vi "Send Count To Caller.vi"(8 "error in (no error)":errorcluster, 10 "Counter":u8, 11 "Counter in":refnum<class "Counter.lvclass">) -> (0 "error out":errorcluster, 3 "Counter out":refnum<class "Counter.lvclass">)   [LabVIEW 2020, in "Counter.lvlib" / "Counter.lvclass"]
uses:
  Counter.lvclass
  C:/Program Files (x86)/National Instruments/LabVIEW 2020/vi.lib/ActorFramework/Actor/Actor.lvclass
  <vilib>/ActorFramework/Actor/Actor.lvclass/Actor.ctl
  Digital Acquisition Messages/Update Data Msg/Update Data Msg.lvclass/Update Data Msg.ctl
  <vilib>/ActorFramework/Message Enqueuer/Message Enqueuer.lvclass/Message Enqueuer.ctl
  <vilib>/ActorFramework/Message Enqueuer/Enqueue.vi
  Digital Acquisition Messages/Update Data Msg/Update Data Msg.lvclass
  C:/Program Files (x86)/National Instruments/LabVIEW 2020/vi.lib/ActorFramework/Message/Message.lvclass
  <vilib>/ActorFramework/Message Priority Queue/Priority Enqueue.vi
  <vilib>/ActorFramework/Actor/Actor.lvclass
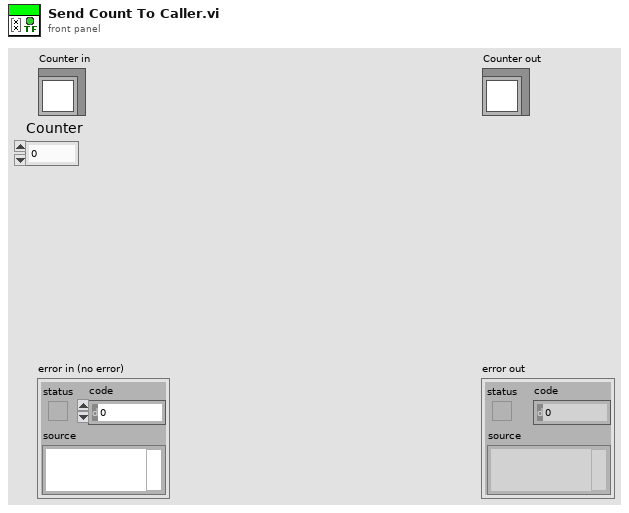
[diagram p1: front panel]
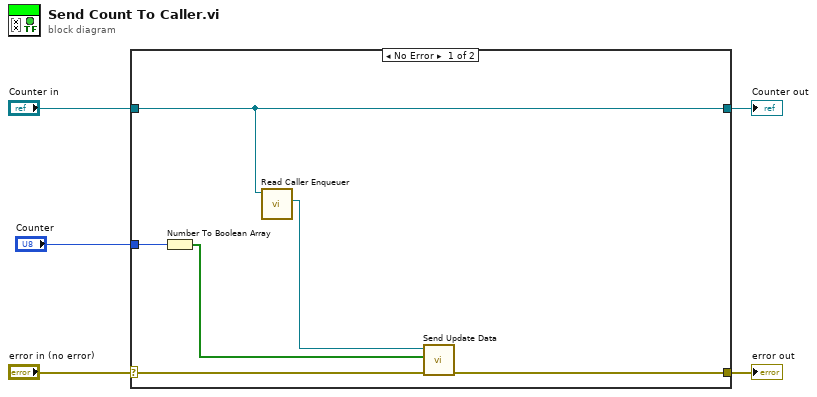
[diagram p0: block diagram]
diagram:
  n1 = case shown="No Error" "error in (no error)" {
    selector: "error in (no error)" -> [w10 w13]
    tunnel: [w9 w13] -> w4
    tunnel: [w11 w12] -> w2
    tunnel: "Counter in" -> [w11 w12]
    tunnel: "Counter" -> [w7 _]
    frame No Error {
      n2 = Number To Boolean Array(number=w7) -> (Boolean array=w6:bool[])
      n3 = call <vilib>:"Read Caller Enqueuer.vi"("Actor"=w11) -> ("Caller Enqueuer"=w8:refnum<class "Message Enqueuer.lvclass">)  [unwired: 10 in]
      n4 = call "Send Update Data.vi"("error in (no error)"=w10, "Data"=w6, "Message Enqueuer"=w8) -> ("error out"=w9:errorcluster)  [unwired: 7 in, 1 out]
    }
    frame Error {
    }
  }
  "error out" <- w4
  "Counter out" <- w2
